vi "UpdateStartFlag.vi"(8 "error in (no error)":errorcluster, 9 "BlkComplete":bool=TRUE, 10 "group":string, 11 "config":variant) -> (0 "error out":errorcluster, 3 "config":variant)   [LabVIEW 2017, in "DataAccumulator.lvlib"]
uses:
  <vilib>/addons/InsightCM/Devices/Shared/Common/DataAccumulator/DataAccumulator.lvlib
  <vilib>/addons/InsightCM/Devices/Shared/Common/DataAccumulator/controls/config.ctl
  <vilib>/addons/InsightCM/Devices/Shared/Common/DeviceHealth/controls/deviceHealthTag.ctl
  <vilib>/addons/InsightCM/Devices/Shared/Common/DeviceHealth/controls/SystemHealthTagEnum.ctl
  <vilib>/addons/InsightCM/MessageBus/Base/controls/Tag.ctl
  <vilib>/addons/InsightCM/MessageBus/Base/controls/KeyValuePair.ctl
  <vilib>/addons/InsightCM/Devices/Shared/Common/DeviceHealth/DeviceHealth.lvlib
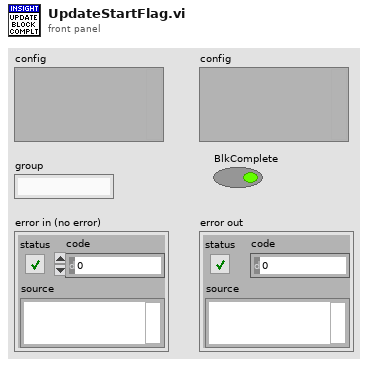
[diagram p1: front panel]
types:
  T1 = typedef "DataAccumulator.lvlib/config.ctl" = cluster{"Group":string, "BlockComplete":bool, "Ok To Start":bool, "Speed Ref Chan":string, "Current OpState":string, "MaxLowRateCPU(%)":dbl, "MaxLowRateMem(%)":dbl, "LowRateCount":i32, "LowRateCountTag":T2}
  T2 = typedef "DeviceHealth.lvlib/deviceHealthTag.ctl" = cluster{"SystemTags":T3, "TagId":string, "Tag":T4}
  T3 = typedef "DeviceHealth.lvlib/SystemHealthTagEnum.ctl" = enum16{"CPU Utilization", "Memory Utilization", "Disk Utilization", "Total Physical Memory", "Primary Disk Free", "Chassis Temperature", "LowRateCount"}
  T4 = typedef "Tag.ctl" = cluster{"Id":string, "Path":string, "Name":string, "Datatype":string, "Props":T5[], "Keywords":string[]}
  T5 = typedef "KeyValuePair.ctl" = cluster{"Key":string, "Value":string}
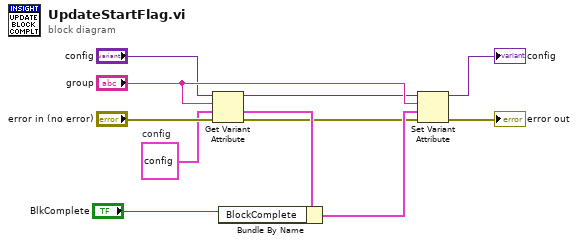
[diagram p0: block diagram]
diagram:
  w6 = T1 {"Group"="", "BlockComplete"=FALSE, "Ok To Start"=FALSE, "Speed Ref Chan"="", "Current OpState"="", "MaxLowRateCPU(%)"=0.0, "MaxLowRateMem(%)"=0.0, "LowRateCount"=0, "LowRateCountTag"={"SystemTags"=enum."CPU Utilization", "TagId"="", "Tag"={"Id"="", "Path"="", "Name"="", "Datatype"="", "Props"=[], "Keywords"=[]}}}  # config
  n1 = Get Variant Attribute(Variant="config", name="group", default value (empty Variant)=w6, error in="error in (no error)") -> (duplicate Variant=w4:variant, value=w7:T1, error out=w2:errorcluster)  [unwired: 1 out]
  n2 = Bundle By Name(cluster=w7, "BlockComplete"="BlkComplete") -> (w8:T1)
  n3 = Set Variant Attribute(Variant=w4, name="group", value=w8, error in=w2) -> (Variant out=→"config":variant, error out=→"error out":errorcluster)  [unwired: 1 out]
